vi "fpga_status.vi"(8 "error in (no error)":errorcluster, 11 "pulse_gen_and_detect_p2p in":refnum<class "pulse_gen_and_detect_p2p.lvclass">) -> (0 "error out":errorcluster, 2 "pulse TX status":T1, 3 "pulse_gen_and_detect_p2p out":refnum<class "pulse_gen_and_detect_p2p.lvclass">)   [LabVIEW 2021, in "pulse_gen_and_detect_p2p.lvclass"]
uses:
  pulse_gen_and_detect_p2p.lvclass
  pulse_gen_and_detect_p2p.lvclass/pulse_gen_and_detect_p2p.ctl
  <vilib>/Utility/error.llb/Error Cluster From Error Code.vi
  <vilib>/rvi/errors/niLvFpgaAdjustHostInterfaceError.vi
  <vilib>/rvi/interface/nirviReadWriteControl/nirviReadWriteControl.xnode
  <vilib>/rvi/interface/nirviMethod/nirviMethod.xnode
  <resource>/objmgr/PeerToPeerStream.rc
  NiFpgaLv.dll
  <vilib>/rvi/interface/Simulation/niFpgaSimulationCallBeginRW.vi
  <vilib>/FPGAPlugInAG/Dynamic/niLvFpga_ReadFifo_Dynamic.vi
  <vilib>/rvi/errors/niLvFpgaMergeErrorWithErrorCode.vi
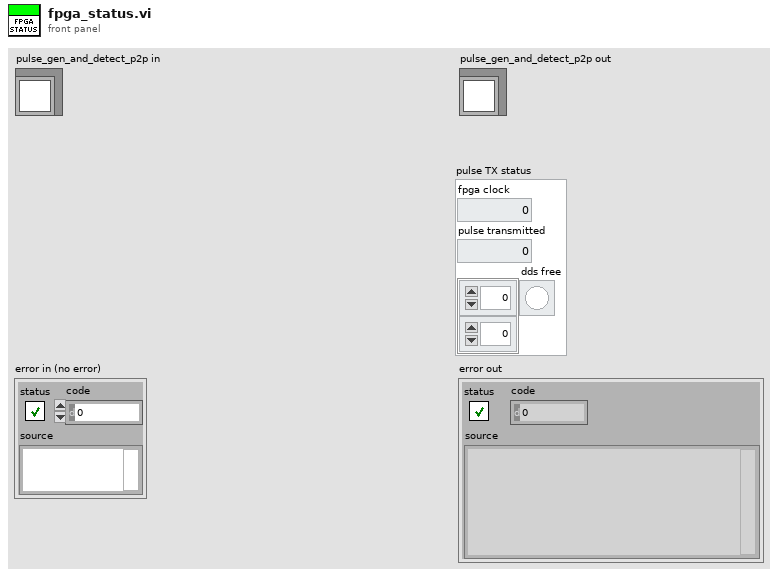
[diagram p1: front panel]
types:
  T1 = cluster{"fpga clock":dbl, "pulse transmitted":u32, "dds free":bool[][]}
  T2 = cluster{"fpga clock":u64, "pulse transmitted":u32, "dds free":bool[]}
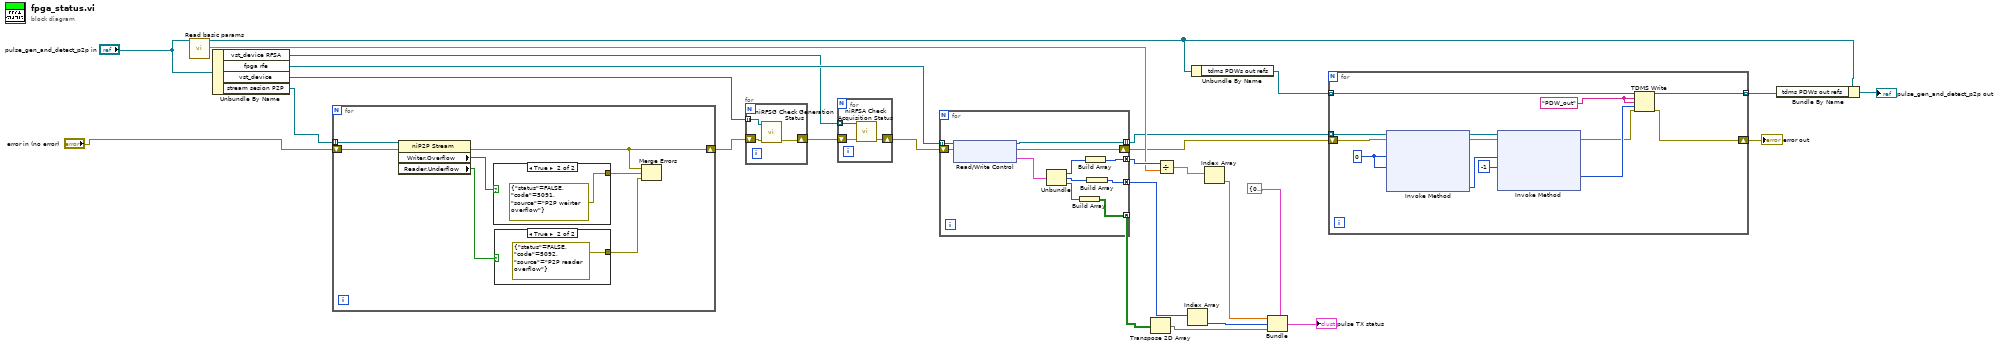
[diagram p0: block diagram]
diagram:
  n1 = call-dynamic "Read basic params.vi"("device_type in"="pulse_gen_and_detect_p2p in") -> ("device_type out"=w3:refnum<class "pulse_gen_and_detect_p2p.lvclass">, "Fs  FPGA"=w23:dbl)  [unwired: 13 in, 4 out]
  n2 = Unbundle By Name("pulse_gen_and_detect_p2p in") -> ("vst_device RFSA"=w8:refnum<k15>[], "fpga rfe"=w25:refnum<k20>[], "vst_device"=w16:refnum<k15>[], "stream sesion P2P"=w14:refnum<k20>[])
  n3 = for {
    shift-right: [w29] -> w15
    shift-left: "error in (no error)" -> [w33]
    tunnel: w14 -> [w32] mode=indexing
    n4 = property class="niP2P Stream"(reference=w32, error in=w33) -> (error out=w29:errorcluster, "Writer.Overflow"=w31:bool, "Reader.Underflow"=w30:bool)  [unwired: 1 out]
    n5 = case shown="True" w31 {
      tunnel: [_ errorcluster {"status"=FALSE, "code"=5091, "source"="P2P weirter overflow"} ("error out")] -> w28
      frame False {
      }
      frame True {
      }
    }
    n6 = case shown="True" w30 {
      tunnel: [_ errorcluster {"status"=FALSE, "code"=5092, "source"="P2P reader overflow"} ("error out")] -> w27
      frame False {
      }
      frame True {
      }
    }
    n7 = Merge Errors(w29, w28, w27) -> ()  [unwired: 1 out]
  }
  n8 = for {
    tunnel: w16 -> [w38] mode=indexing
    shift-right: [w36] -> w10
    shift-left: w15 -> [w37]
    n9 = call <instrlib>:"niRFSG Check Generation Status.vi"("instrument handle"=w38, "error in"=w37) -> ("error out"=w36:errorcluster)  [unwired: 11 in, 2 out]
  }
  n10 = for {
    tunnel: w8 -> [w39] mode=indexing
    shift-right: [w40] -> w9
    shift-left: w10 -> [w41]
    n11 = call <instrlib>:"niRFSA Check Acquisition Status.vi"("instrument handle"=w39, "error in"=w41) -> ("error out"=w40:errorcluster)  [unwired: 11 in, 2 out]
  }
  n12 = for {
    tunnel: w25 -> [w49] mode=indexing
    shift-right: [w51] -> w6
    shift-left: w9 -> [w52]
    tunnel: [w50] -> w7 mode=indexing
    tunnel: [w48] -> w24 mode=concatenating
    tunnel: [w47] -> w19 mode=concatenating
    tunnel: [w46] -> w26 mode=concatenating
    n13 = xnode "Read/Write Control"("FPGA VI Reference In"=w49, "error in"=w52) -> ("FPGA VI Reference Out"=w50:refnum<k20>, "error out"=w51:errorcluster, "pulse TX status"=w45:T2)
    n14 = Unbundle(w45) -> ("fpga clock"=w44:u64, "pulse transmitted"=w43:u32, "dds free"=w42:bool[])
    n15 = Build Array(w42) -> (w48:bool[][])
    n16 = Build Array(w44) -> (w46:u64[])
    n17 = Build Array(w43) -> (w47:u32[])
  }
  n18 = Transpose 2D Array(2D array=w24) -> (transposed array=w22:bool[][])
  n19 = Divide(x=w26, y=w23) -> (x/y=w21:dbl[])
  n20 = Index Array(array=w19) -> (element=w18:u32)  [unwired: 1 in]
  n21 = Unbundle By Name(w3) -> ("tdms PDWs out refs"=w2:refnum<k34>[])
  n22 = Index Array(array=w21) -> (element=w20:dbl)  [unwired: 1 in]
  n23 = Bundle(cluster=T1 {"fpga clock"=0.0, "pulse transmitted"=0, "dds free"=[[FALSE, FALSE, FALSE, FALSE, FALSE, FALSE, FALSE, FALSE, FALSE, FALSE, FALSE, FALSE, FALSE, FALSE, FALSE, FALSE]]} ("pulse TX status"), "fpga clock"=w20, "pulse transmitted"=w18, "dds free"=w22) -> (→"pulse TX status":T1)
  n24 = for {
    tunnel: w7 -> [w65] mode=indexing
    shift-right: [w54] -> w5
    shift-left: w6 -> [w64]
    tunnel: w2 -> [w58] mode=indexing
    tunnel: [w57] -> w1 mode=indexing
    w53 = "PDW_out" ("group name")
    w60 = u32 0 ("Number of Elements")
    n25 = xnode "Invoke Method"("FPGA VI Reference In"=w65, "error in"=w64, "Number of Elements"=w60, "Timeout (ms)"=w60) -> ("FPGA VI Reference Out"=w62:refnum<k20>, "error out"=w63:errorcluster, "Elements Remaining"=w61:u32)  [unwired: 1 out]
    n26 = xnode "Invoke Method"("FPGA VI Reference In"=w62, "error in"=w63, "Number of Elements"=w61, "Timeout (ms)"=-1) -> ("error out"=w55:errorcluster, "Data"=w56:u64[])  [unwired: 2 out]
    n27 = TDMS Write(0:w58, 5:w53, 7:w53, 9:w56, 11:w55) -> (4:w57:refnum<k34>, 15:w54:errorcluster)  [unwired: 1 in, 2 out]
  }
  "error out" <- w5
  n28 = Bundle By Name(cluster=w3, "tdms PDWs out refs"=w1) -> (→"pulse_gen_and_detect_p2p out":refnum<class "pulse_gen_and_detect_p2p.lvclass">)
